vi "openCamera.vi"(0 "error in":errorcluster, 2 "Camera Settings":T2={"Camera"=enum."left_hand_camera", "FPS"=20.0, "Camera Controls"=[], "Resolution"=enum."(320, 200)"}, 3 "node":string) -> (1 "error out":errorcluster, 4 "Error Code":i32)   [LabVIEW 2013]
doc: "Opens a connection to a Baxter Camera"
uses:
  ROS/Code/SubVIs/BaxterCamera.ctl
panel:
  out "Reply":string
  out "OK?":bool
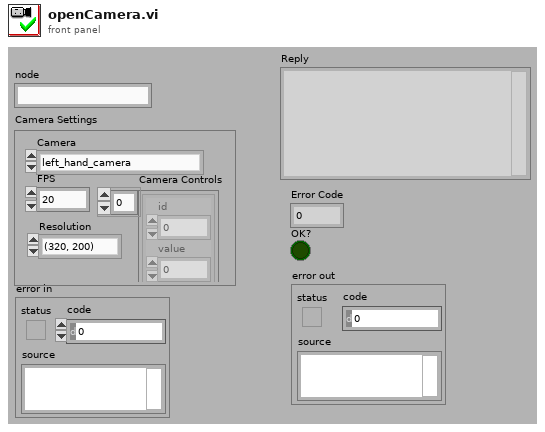
[diagram p1: front panel]
types:
  T1 = typedef "BaxterCamera.ctl" = enum16{"left_hand_camera", "right_hand_camera", "head_camera"}
  T2 = cluster{"Camera":T1, "FPS":sgl, "Camera Controls":cluster{"id":i32, "value":i32}[], "Resolution":enum16{"(1280, 800)", "(960, 600)", "(640, 400)", "(480, 300)", "(384, 240)", "(320, 200)"}}
  T3 = typedef "_ROSControl.ctl" = cluster{"topic port":u16, "Node":string, "topic":string, "type":string, "node port":u32, "error ":errorcluster, "Direction":T4, "APIs":string[]}
  T4 = typedef "_ROSDirection.ctl" = enum16{"Node", "Publisher", "Subscriber", "Service Client"}
  T5 = enum16{"(1280, 800)", "(960, 600)", "(640, 400)", "(480, 300)", "(384, 240)", "(320, 200)"}
  T6 = cluster{string, "FPS":sgl, "Camera Controls":cluster{"id":i32, "value":i32}[], "Resolution":enum16{"(1280, 800)", "(960, 600)", "(640, 400)", "(480, 300)", "(384, 240)", "(320, 200)"}}
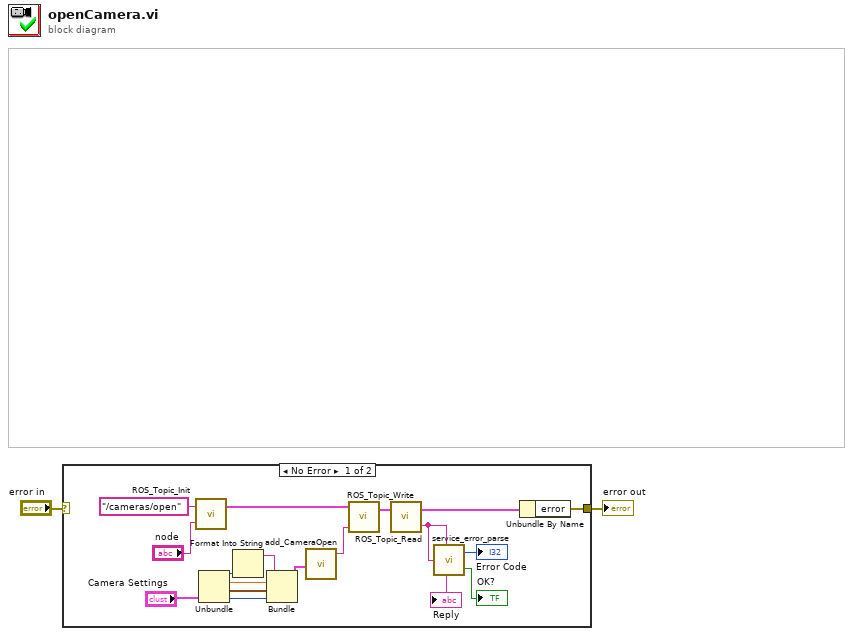
[diagram p0: block diagram]
diagram:
  n1 = case shown="No Error" "error in" {
    selector: "error in" -> [_ w20]
    tunnel: [w19 w20] -> w2
    frame No Error {
      n2 = call "ROS_Topic_Init.vi"("node"="node", "topic"="/cameras/open") -> ("ROS out"=w17:T3)  [unwired: 1 in]
      n3 = Unbundle("Camera Settings") -> ("Camera"=w5:T1, "FPS"=w6:sgl, "Camera Controls"=w7:cluster{"id":i32, "value":i32}[], "Resolution"=w8:T5)
      n4 = Format Into String(w5) -> (resulting string=w4:string)  [unwired: 3 in, 1 out]
      n5 = Bundle(w4, "FPS"=w6, "Camera Controls"=w7, "Resolution"=w8) -> (w3:T6)  [unwired: 1 in]
      n6 = call "add_CameraOpen.vi"("Camera Settings"=w3) -> ("msg out"=w13:string)  [unwired: 4 in]
      n7 = call "ROS_Topic_Write.vi"("Msg in"=w13, "ROS in"=w17) -> ("ROS out"=w15:T3)  [unwired: 2 in]
      n8 = call "ROS_Topic_Read.vi"("ROS in"=w15) -> ("Reply"=w12:string, "ROS out"=w14:T3)  [unwired: 1 in]
      "Reply" <- w12
      n9 = call "service_error_parse.vi"("Reply"=w12) -> ("OK?"=→"OK?":bool, "Error Code"=→"Error Code":i32)
      n10 = Unbundle By Name(w14) -> ("error"=w19:errorcluster)
    }
    frame Error {
    }
  }
  "error out" <- w2
